vi "APC_WarningBool.vi"(2 "CylPresErrors":u64, 3 "CylPresWarnings":u64) -> (0 "Error":bool[][](array[boolean]), 1 "Warning":bool[][](array[boolean]))   [LabVIEW 2020]
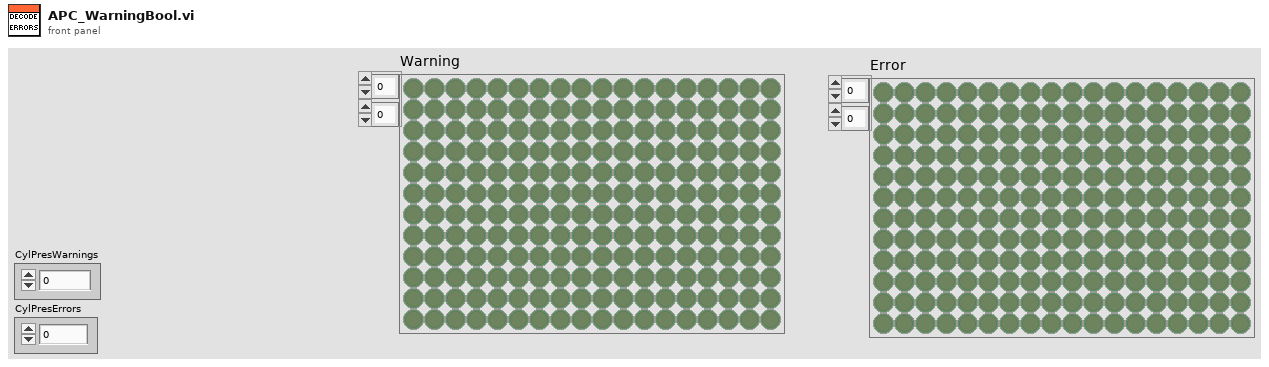
[diagram p1: front panel]
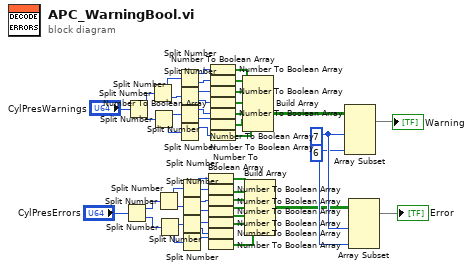
[diagram p0: block diagram]
diagram:
  w5 = 6 ("length")
  w6 = 7 ("length")
  n1 = Split Number(x="CylPresErrors") -> (hi(x)=w27:u32, lo(x)=w26:u32)
  n2 = Split Number(x="CylPresWarnings") -> (hi(x)=w47:u32, lo(x)=w46:u32)
  n3 = Split Number(x=w47) -> (hi(x)=w45:u16, lo(x)=w44:u16)
  n4 = Split Number(x=w46) -> (hi(x)=w43:u16, lo(x)=w42:u16)
  n5 = Split Number(x=w27) -> (hi(x)=w25:u16, lo(x)=w24:u16)
  n6 = Split Number(x=w26) -> (hi(x)=w23:u16, lo(x)=w22:u16)
  n7 = Split Number(x=w45) -> (hi(x)=w41:u8, lo(x)=w40:u8)
  n8 = Split Number(x=w44) -> (hi(x)=w39:u8, lo(x)=w38:u8)
  n9 = Split Number(x=w43) -> (hi(x)=w37:u8, lo(x)=w36:u8)
  n10 = Split Number(x=w42) -> (hi(x)=w35:u8)  [unwired: 1 out]
  n11 = Split Number(x=w25) -> (hi(x)=w21:u8, lo(x)=w20:u8)
  n12 = Split Number(x=w24) -> (hi(x)=w19:u8, lo(x)=w18:u8)
  n13 = Split Number(x=w23) -> (hi(x)=w17:u8, lo(x)=w16:u8)
  n14 = Split Number(x=w22) -> (hi(x)=w15:u8)  [unwired: 1 out]
  n15 = Number To Boolean Array(number=w21) -> (Boolean array=w14:bool[])
  n16 = Number To Boolean Array(number=w20) -> (Boolean array=w13:bool[])
  n17 = Number To Boolean Array(number=w19) -> (Boolean array=w12:bool[])
  n18 = Number To Boolean Array(number=w18) -> (Boolean array=w11:bool[])
  n19 = Number To Boolean Array(number=w17) -> (Boolean array=w10:bool[])
  n20 = Number To Boolean Array(number=w16) -> (Boolean array=w9:bool[])
  n21 = Number To Boolean Array(number=w15) -> (Boolean array=w8:bool[])
  n22 = Number To Boolean Array(number=w41) -> (Boolean array=w34:bool[])
  n23 = Number To Boolean Array(number=w40) -> (Boolean array=w33:bool[])
  n24 = Number To Boolean Array(number=w39) -> (Boolean array=w32:bool[])
  n25 = Number To Boolean Array(number=w38) -> (Boolean array=w31:bool[])
  n26 = Number To Boolean Array(number=w37) -> (Boolean array=w30:bool[])
  n27 = Number To Boolean Array(number=w36) -> (Boolean array=w29:bool[])
  n28 = Number To Boolean Array(number=w35) -> (Boolean array=w28:bool[])
  n29 = Build Array(w34, w33, w32, w31, w30, w29, w28) -> (w4:bool[][])
  n30 = Build Array(w14, w13, w12, w11, w10, w9, w8) -> (w2:bool[][])
  n31 = Array Subset(array=w4, length (row)=w6, length (col)=w5) -> (→"Warning":bool[][])  [unwired: 2 in]
  n32 = Array Subset(array=w2, length (row)=w6, length (col)=w5) -> (→"Error":bool[][])  [unwired: 2 in]
